vi "IRAlg.vi"(9 "Stabilize":T2(ring), 10 "IRValIn":dbl[](array[numeric]), 11 "Cluster":T1) -> (1 "VelValOut":dbl[](array[numeric]), 2 "logical AND":bool, 3 "0, 1":i16)   [LabVIEW 2019]
uses:
  <vilib>/functionblocks/Counter/Count Up/Count Up.vi
  <vilib>/functionblocks/FB Core/FB Core.xnode
  <vilib>/functionblocks/NI_FunctionBlock Libraries.lvlib
panel:
  out "OU":dbl
  out "X":dbl
  out "Y":dbl
  out "Sense":dbl
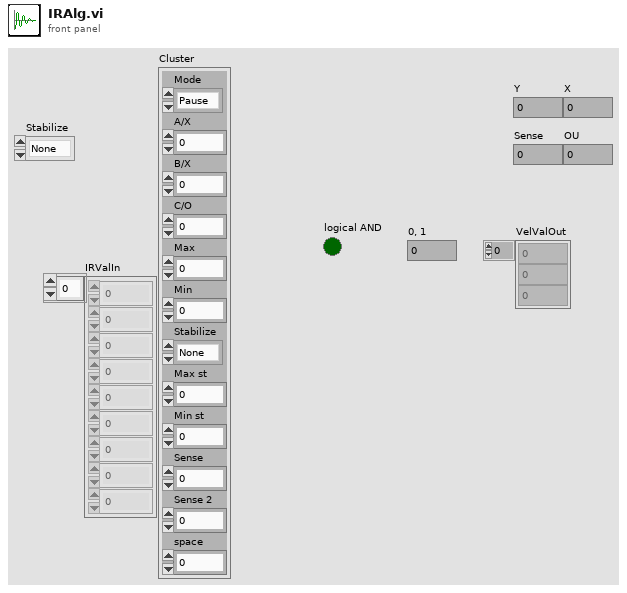
[diagram p1: front panel]
types:
  T1 = cluster{"Mode":enum16{"Pause", "Encoder", "Stabilized"}, "A/X":dbl, "B/X":dbl, "C/O":dbl, "Max":dbl, "Min":dbl, "Stabilize":enum16{"None", "Wall Left", "Wall Right", "Wall Front & Line", "Wall Rear & Left", "Wall Rear & Right", "Wall Rear", "Line", "Wall Front", "Wall Front & Left", "Wall Front & Right"}, "Max st":dbl, "Min st":dbl, "Sense":dbl, "Sense 2":dbl, "space":dbl}
  T2 = enum16{"None", "Wall Left", "Wall Right", "Wall Front & Line", "Wall Rear & Left", "Wall Rear & Right", "Wall Rear", "Line", "Wall Front", "Wall Front & Left", "Wall Front & Right"}
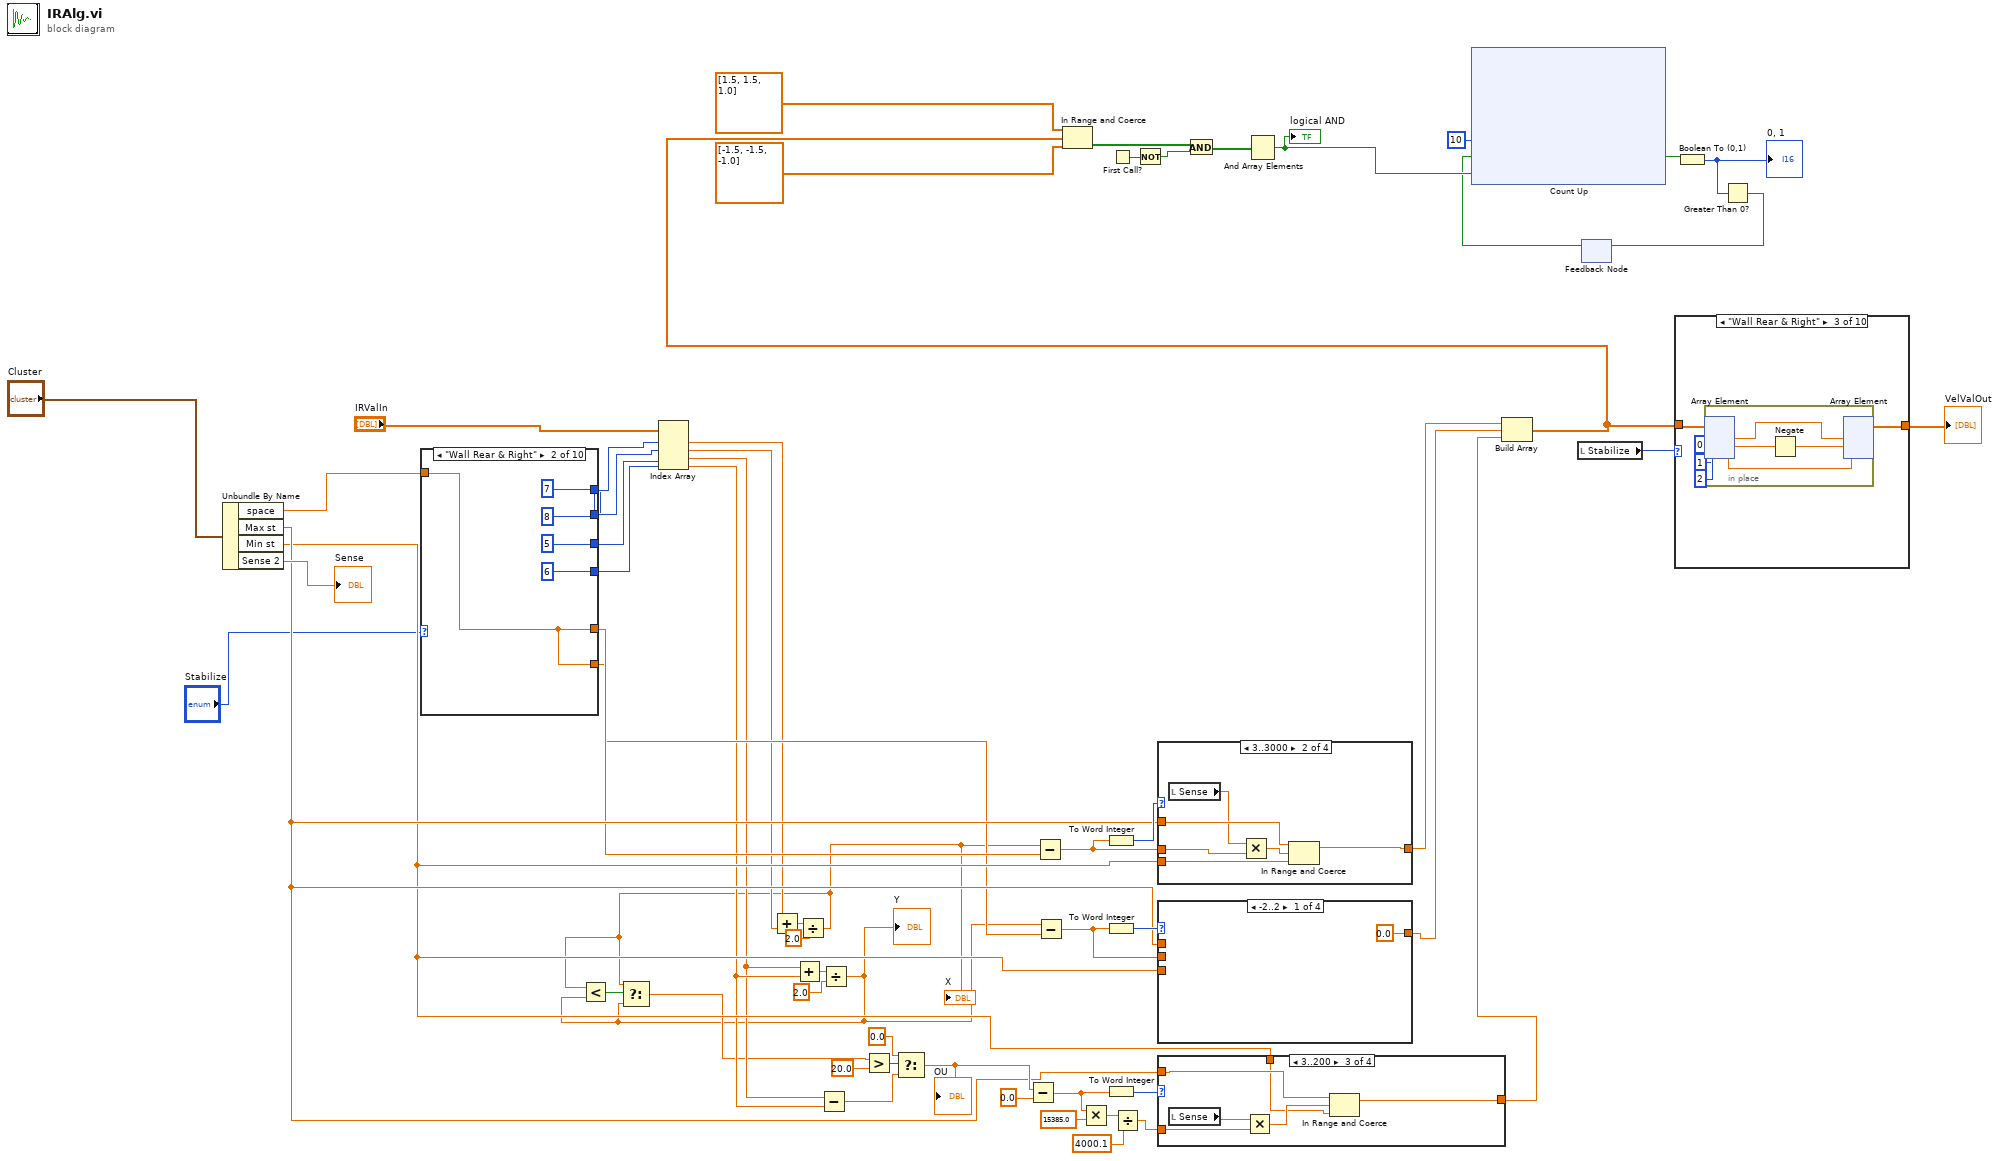
[diagram p0: block diagram]
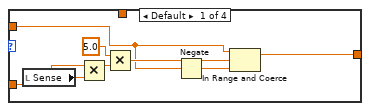
[diagram p2: hidden frame]
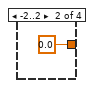
[diagram p3: hidden frame]
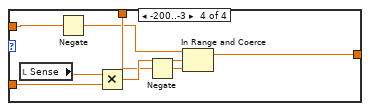
[diagram p4: hidden frame]
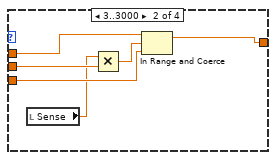
[diagram p5: hidden frame]
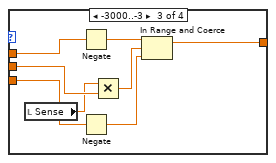
[diagram p6: hidden frame]
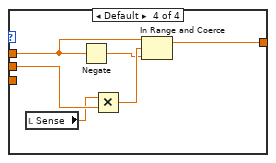
[diagram p7: hidden frame]
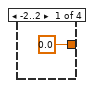
[diagram p8: hidden frame]
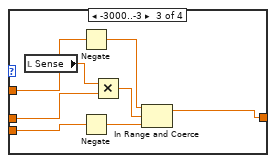
[diagram p9: hidden frame]
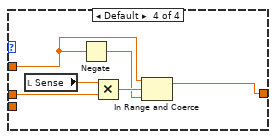
[diagram p10: hidden frame]
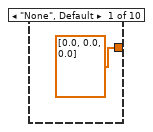
[diagram p11: hidden frame]
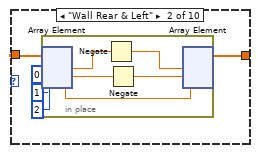
[diagram p12: hidden frame]
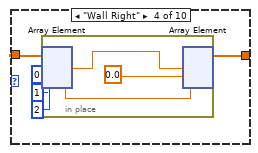
[diagram p13: hidden frame]
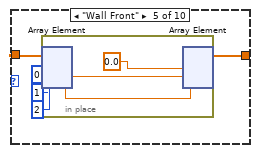
[diagram p14: hidden frame]
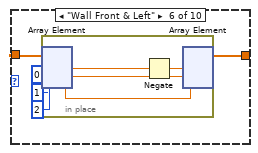
[diagram p15: hidden frame]
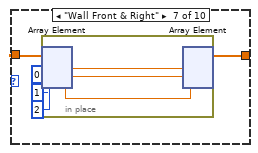
[diagram p16: hidden frame]
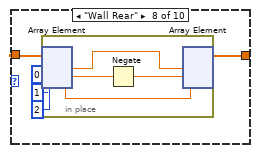
[diagram p17: hidden frame]
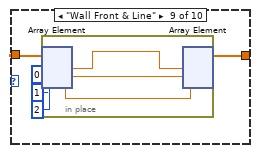
[diagram p18: hidden frame]
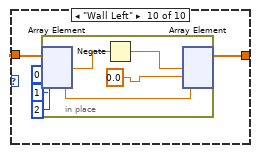
[diagram p19: hidden frame]
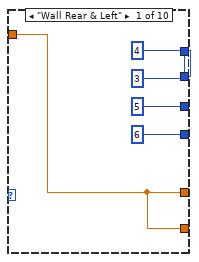
[diagram p20: hidden frame]
diagram:
  n1 = Unbundle By Name("Cluster") -> ("space"=w50:dbl, "Max st"=w30:dbl, "Min st"=w29:dbl, "Sense 2"=→"Sense":dbl)
  n2 = case shown="\"Wall Rear & Right\"" "Stabilize" {
    tunnel: [4 7 7 3 0 0 0 4 8 0] -> w23
    tunnel: [3 8 8 4 0 0 0 3 7 0] -> w24
    tunnel: [5 5 3 8 0 1 1 1 1 5] -> w22
    tunnel: [6 6 4 7 0 1 1 1 1 6] -> w21
    tunnel: [w60 w65 w70 w75 0.0 ("space") 0.0 ("space") 0.0 ("space") w98 w103 0.0 ("space")] -> w27
    tunnel: w50 -> [w60 w65 w70 w75 _ w87 w93 w98 w103 w109]
    tunnel: [w60 w65 w70 w75 0.0 ("space") w87 w93 w98 w103 w109] -> w26
    frame "Wall Rear & Left" {
    }
    frame "Wall Rear & Right" {
    }
    frame "Wall Right" {
    }
    frame "Wall Left" {
    }
    frame Default {
    }
    frame "Wall Front & Line" {
    }
    frame "Wall Front" {
    }
    frame "Wall Front & Left" {
    }
    frame "Wall Front & Right" {
    }
    frame "Wall Rear" {
    }
  }
  n3 = Index Array(array="IRValIn", index #1=w24, index #2=w23, index #3=w22, index #4=w21) -> (element #1=w17:dbl, element #2=w18:dbl, element #3=w19:dbl, element #4=w20:dbl)
  n4 = Add(x=w17, y=w18) -> (x+y=w45:dbl)
  n5 = Add(x=w19, y=w20) -> (x+y=w46:dbl)
  n6 = Divide(x=w45, y=2.0) -> (x/y=w11:dbl)
  "X" <- w11
  n7 = Subtract(x=w19, y=w20) -> (x-y=w48:dbl)
  n8 = Divide(x=w46, y=2.0) -> (x/y=w10:dbl)
  "Y" <- w10
  n9 = Less?(x=w11, y=w10) -> (x < y?=w13:bool)
  n10 = Select(t=w11, s=w13, f=w10) -> (s? t:f=w12:dbl)
  n11 = Greater?(x=w12, y=20.0) -> (0:w47:bool)
  n12 = Select(t=0.0, s=w47, f=w48) -> (s? t:f=w49:dbl)
  "OU" <- w49
  n13 = Subtract(x=w49, y=0.0) -> (x-y=w43:dbl)
  n14 = Subtract(x=w11, y=w27) -> (x-y=w40:dbl)
  n15 = Subtract(x=w10, y=w26) -> (x-y=w41:dbl)
  n16 = Multiply(x=w43, y=15385.0) -> (x*y=w42:dbl)
  n17 = To Word Integer(number=w40) -> (16bit integer=w39:i16)
  n18 = To Word Integer(number=w41) -> (16bit integer=w38:i16)
  n19 = To Word Integer(number=w43) -> (16bit integer=w37:i16)
  n20 = First Call?() -> (First Call?: T/F=w56:bool)
  n21 = Divide(x=w42, y=4000.1) -> (x/y=w44:dbl)
  n22 = Not(x=w56) -> (.not. x?=w55:bool)
  n23 = case shown="3..3000" w39 {
    tunnel: w40 -> [_ w118 w126 w132]
    tunnel: [0.0 ("x") w119 w127 w133] -> w16
    tunnel: w30 -> [_ w117 w125 w131]
    tunnel: w29 -> [_ w116 w123 _]
    frame -2..2 {
    }
    frame 3..3000 {
      n24 = local read "Sense"() -> (w115:dbl)
      n25 = Multiply(x=w115, y=w118) -> (x*y=w120:dbl)
      n26 = In Range and Coerce(upper limit=w117, x=w120, lower limit=w116) -> (coerced(x)=w119:dbl)  [unwired: 1 out]
    }
    frame -3000..-3 {
      n27 = local read "Sense"() -> (w121:dbl)
      n28 = Negate(x=w125) -> (-x=w122:dbl)
      n29 = Negate(x=w123) -> (-x=w124:dbl)
      n30 = Multiply(x=w121, y=w126) -> (x*y=w128:dbl)
      n31 = In Range and Coerce(upper limit=w122, x=w128, lower limit=w124) -> (coerced(x)=w127:dbl)  [unwired: 1 out]
    }
    frame Default {
      n32 = local read "Sense"() -> (w129:dbl)
      n33 = Negate(x=w131) -> (-x=w130:dbl)
      n34 = Multiply(x=w129, y=w132) -> (x*y=w134:dbl)
      n35 = In Range and Coerce(upper limit=w131, x=w134, lower limit=w130) -> (coerced(x)=w133:dbl)  [unwired: 1 out]
    }
  }
  n36 = case shown="-2..2" w38 {
    tunnel: w41 -> [_ w139 w147 w153]
    tunnel: [0.0 ("x") w140 w148 w154] -> w15
    tunnel: w30 -> [_ w138 w143 w151]
    tunnel: w29 -> [_ w137 w144 _]
    frame -2..2 {
    }
    frame 3..3000 {
      n37 = local read "Sense"() -> (w136:dbl)
      n38 = Multiply(x=w136, y=w139) -> (x*y=w141:dbl)
      n39 = In Range and Coerce(upper limit=w138, x=w141, lower limit=w137) -> (coerced(x)=w140:dbl)  [unwired: 1 out]
    }
    frame -3000..-3 {
      n40 = local read "Sense"() -> (w142:dbl)
      n41 = Negate(x=w143) -> (-x=w146:dbl)
      n42 = Negate(x=w144) -> (-x=w145:dbl)
      n43 = Multiply(x=w142, y=w147) -> (x*y=w149:dbl)
      n44 = In Range and Coerce(upper limit=w146, x=w149, lower limit=w145) -> (coerced(x)=w148:dbl)  [unwired: 1 out]
    }
    frame Default {
      n45 = local read "Sense"() -> (w150:dbl)
      n46 = Negate(x=w151) -> (-x=w152:dbl)
      n47 = Multiply(x=w150, y=w153) -> (x*y=w155:dbl)
      n48 = In Range and Coerce(upper limit=w151, x=w155, lower limit=w152) -> (coerced(x)=w154:dbl)  [unwired: 1 out]
    }
  }
  n49 = case shown="3..200" w37 {
    tunnel: w44 -> [w160 _ w168 w176]
    tunnel: [w161 0.0 ("x") w169 w177] -> w14
    tunnel: w30 -> [w156 _ w166 w174]
    tunnel: w29 -> [_ _ w165 w173]
    frame Default {
      n50 = local read "Sense"() -> (w158:dbl)
      n51 = Multiply(x=w160, y=w158) -> (x*y=w159:dbl)
      n52 = Multiply(x=5.0, y=w159) -> (x*y=w163:dbl)
      n53 = Negate(x=w156) -> (-x=w157:dbl)
      n54 = In Range and Coerce(upper limit=w156, x=w163, lower limit=w157) -> (coerced(x)=w161:dbl)  [unwired: 1 out]
    }
    frame -2..2 {
    }
    frame 3..200 {
      n55 = local read "Sense"() -> (w167:dbl)
      n56 = Multiply(x=w167, y=w168) -> (x*y=w170:dbl)
      n57 = In Range and Coerce(upper limit=w166, x=w170, lower limit=w165) -> (coerced(x)=w169:dbl)  [unwired: 1 out]
    }
    frame -200..-3 {
      n58 = local read "Sense"() -> (w175:dbl)
      n59 = Negate(x=w174) -> (-x=w172:dbl)
      n60 = Multiply(x=w175, y=w176) -> (x*y=w178:dbl)
      n61 = Negate(x=w173) -> (-x=w171:dbl)
      n62 = In Range and Coerce(upper limit=w172, x=w178, lower limit=w171) -> (coerced(x)=w177:dbl)  [unwired: 1 out]
    }
  }
  n63 = Build Array(w16, w15, w14) -> (w9:dbl[])
  n64 = In Range and Coerce(upper limit=dbl[] [1.5, 1.5, 1.0], x=w9, lower limit=dbl[] [-1.5, -1.5, -1.0]) -> (In Range?=w57:bool[])  [unwired: 1 out]
  n65 = And(x=w57, y=w55) -> (x .and. y?=w54:bool[])
  n66 = And Array Elements(Boolean array=w54) -> (logical AND=w5:bool)
  "logical AND" <- w5
  n67 = local read "Stabilize"() -> (w51:T2)
  n68 = feedback #1() -> (w1:bool)  [unwired: 1 in]
  n69 = xnode "Count Up"("preset value"=u32 10, "reset"=w1, "count up"=w5) -> ("done"=w6:bool)  [unwired: 1 in, 2 out]
  n70 = case shown="\"Wall Rear & Right\"" w51 {
    tunnel: [dbl[] [0.0, 0.0, 0.0] ("IRValIn") w181 w191 w200 w208 w216 w225 w233 w242 w250] -> w52
    tunnel: w9 -> [_ w180 w190 w199 w207 w215 w224 w232 w241 w249]
    frame "None", Default {
    }
    frame "Wall Rear & Left" {
      n71 = in-place {
        n72 = in-place-array #2(w180, 0, 1, 2) -> (w189:dbl, w188:dbl, w187:dbl)
        n73 = Negate(x=w189) -> (-x=w185:dbl)
        n74 = Negate(x=w188) -> (-x=w186:dbl)
        n75 = in-place-array #2(w185, w186, w187) -> (w181:dbl[])  [unwired: 3 out]
      }
    }
    frame "Wall Rear & Right" {
      n76 = in-place {
        n77 = in-place-array #3(w190, 0, 1, 2) -> (w195:dbl, w198:dbl, w197:dbl)
        n78 = Negate(x=w198) -> (-x=w196:dbl)
        n79 = in-place-array #3(w195, w196, w197) -> (w191:dbl[])  [unwired: 3 out]
      }
    }
    frame "Wall Right" {
      n80 = in-place {
        n81 = in-place-array #4(w199, 0, 1, 2) -> (w205:dbl, w206:dbl)  [unwired: 1 out]
        n82 = in-place-array #4(w205, 0.0 ("space"), w206) -> (w200:dbl[])  [unwired: 3 out]
      }
    }
    frame "Wall Front" {
      n83 = in-place {
        n84 = in-place-array #5(w207, 0, 1, 2) -> (w212:dbl, w214:dbl)  [unwired: 1 out]
        n85 = in-place-array #5(0.0 ("space"), w212, w214) -> (w208:dbl[])  [unwired: 3 out]
      }
    }
    frame "Wall Front & Left" {
      n86 = in-place {
        n87 = in-place-array #6(w215, 0, 1, 2) -> (w221:dbl, w222:dbl, w223:dbl)
        n88 = Negate(x=w221) -> (-x=w220:dbl)
        n89 = in-place-array #6(w220, w222, w223) -> (w216:dbl[])  [unwired: 3 out]
      }
    }
    frame "Wall Front & Right" {
      n90 = in-place {
        n91 = in-place-array #7(w224, 0, 1, 2) -> (w229:dbl, w230:dbl, w231:dbl)
        n92 = in-place-array #7(w229, w230, w231) -> (w225:dbl[])  [unwired: 3 out]
      }
    }
    frame "Wall Rear" {
      n93 = in-place {
        n94 = in-place-array #8(w232, 0, 1, 2) -> (w237:dbl, w240:dbl, w239:dbl)
        n95 = Negate(x=w240) -> (-x=w238:dbl)
        n96 = in-place-array #8(w237, w238, w239) -> (w233:dbl[])  [unwired: 3 out]
      }
    }
    frame "Wall Front & Line" {
      n97 = in-place {
        n98 = in-place-array #9(w241, 0, 1, 2) -> (w247:dbl, w246:dbl, w248:dbl)
        n99 = in-place-array #9(w247, w246, w248) -> (w242:dbl[])  [unwired: 3 out]
      }
    }
    frame "Wall Left" {
      n100 = in-place {
        n101 = in-place-array #10(w249, 0, 1, 2) -> (w256:dbl, w257:dbl)  [unwired: 1 out]
        n102 = Negate(x=w256) -> (-x=w255:dbl)
        n103 = in-place-array #10(w255, 0.0 ("space"), w257) -> (w250:dbl[])  [unwired: 3 out]
      }
    }
  }
  "VelValOut" <- w52
  n104 = Boolean To (0,1)(Boolean=w6) -> (0, 1=w3:i16)
  "0, 1" <- w3
  n105 = Greater Than 0?(x=w3) -> (x > 0?=w2:bool)
  n106 = feedback-in #1(w2) -> ()
